vi "DET_get_Data_corrected.vi"(8 "error in (no error)":errorcluster, 10 "Control IN":T1={"# scans"=0, "All"=FALSE, "Parameters of measurement"={"ODmin"=0.0, "ODmax"=0.0, "Aq contol"=enum."fixed", "Wavelength_fix_index"=640, "WCM_limits"={"WCM_min"=0.0, "WCM_max"=0.0, "WCM_value"=0.0}, "WCM_corrections"=FALSE, "#cycles max"=5}}, 11 "Detector in":refnum<class "Detector.lvclass">) -> (0 "error out":errorcluster, 1 "II channel seq":cluster{"BG":i32[], "Ie":i32[], "I0":i32[]}[](array[cluster]), 2 "I channel seq":cluster{"BG":i32[], "Ie":i32[], "I0":i32[]}[](array[cluster]), 3 "Detector out":refnum<class "Detector.lvclass">, 5 "WCM_correction_coff":sgl[](array[numeric]))   [LabVIEW 2015, in "Detector.lvclass"]
uses:
  Detector.lvclass
  dependecies/ControlsVIs/Clusters-def/Det-Read.ctl
  dependecies/ControlsVIs/Clusters-def/Parameters_measurement_def.ctl
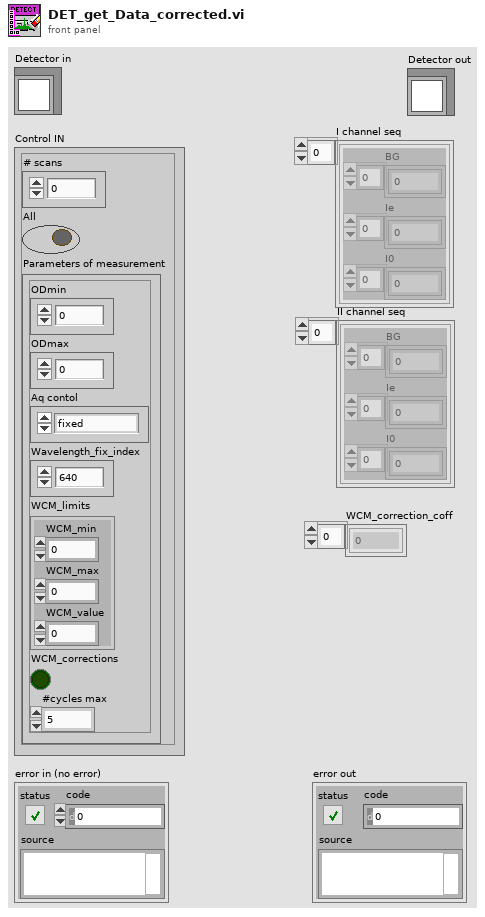
[diagram p1: front panel]
types:
  T1 = typedef "Detector.lvclass/Det-Read.ctl" = cluster{"# scans":i32, "All":bool, "Parameters of measurement":T2}
  T2 = typedef "Parameters_measurement_def.ctl" = cluster{"ODmin":dbl, "ODmax":dbl, "Aq contol":enum32{"fixed", "automatic", "fixed-auto"}, "Wavelength_fix_index":i32, "WCM_limits":cluster{"WCM_min":dbl, "WCM_max":dbl, "WCM_value":dbl}, "WCM_corrections":bool, "#cycles max":i32}
  T3 = cluster{"WCM_min":dbl, "WCM_max":dbl, "WCM_value":dbl}
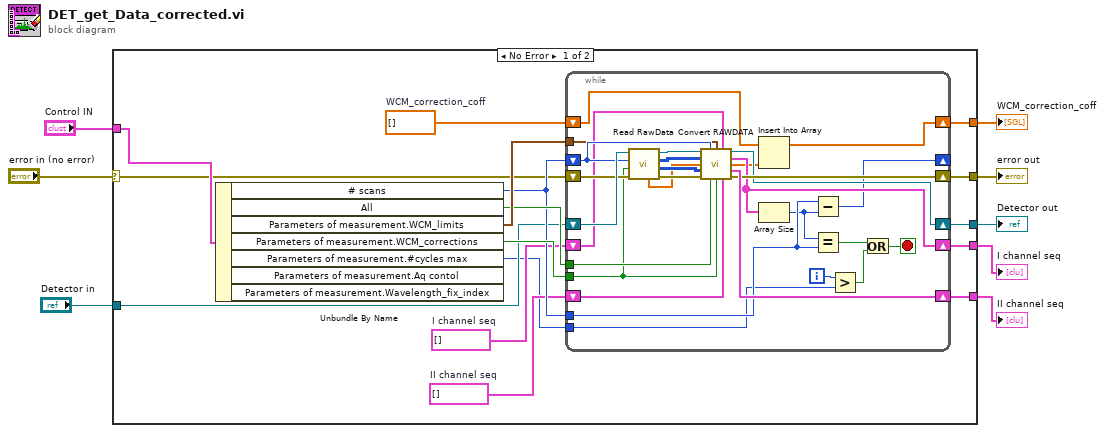
[diagram p0: block diagram]
diagram:
  n1 = case shown="No Error" "error in (no error)" {
    selector: "error in (no error)" -> [w10 w54]
    tunnel: [w18 _] -> w8
    tunnel: [w16 w53] -> w7
    tunnel: [w15 w54] -> w6
    tunnel: [w14 _] -> w5
    tunnel: [w13 _] -> w4
    tunnel: "Detector in" -> [w12 w53]
    tunnel: "Control IN" -> [w11 _]
    frame No Error {
      w20 = cluster{"BG":i32[], "Ie":i32[], "I0":i32[]}[] []  # II channel seq
      w19 = cluster{"BG":i32[], "Ie":i32[], "I0":i32[]}[] []  # I channel seq
      w17 = sgl[] []  # WCM_correction_coff
      n2 = Unbundle By Name(w11) -> ("# scans"=w21:i32, "All"=w22:bool, "Parameters of measurement.WCM_limits"=w23:T3, "Parameters of measurement.WCM_corrections"=w24:bool, "Parameters of measurement.#cycles max"=w9:i32)  [unwired: 2 out]
      n3 = while {
        shift-right: [w45] -> w16
        shift-left: w12 -> [w52]
        shift-right: [w46] -> w15
        shift-left: w10 -> [w44]
        shift-right: [w29] -> w18
        shift-left: w17 -> [w27]
        shift-right: [w40] -> w13
        shift-left: w19 -> [w42]
        shift-right: [w47] -> w14
        shift-left: w20 -> [w41]
        shift-right: [w33] -> _
        shift-left: w21 -> [w43]
        tunnel: w21 -> [w35]
        tunnel: w22 -> [w32]
        tunnel: w23 -> [w31]
        tunnel: w24 -> [w26]
        tunnel: w9 -> [w25]
        i -> [w39]
        stop <- w36 stop-if-true
        n4 = call-dynamic "Read RawData.vi"("error in (no error)"=w44, "WCM_max_value"=w26, "# of scans"=w43, "Detector in"=w52) -> ("error out"=w50:errorcluster, "Channel II"=w48:i32[][], "Channel I"=w49:i32[][], "Detector out"=w51:refnum<class "Detector.lvclass">, "WCM_values"=w30:sgl[])  [unwired: 3 in]
        n5 = call-dynamic "Convert RAWDATA.vi"("Detector in"=w51, "# of scan"=w43, "WCM_limits"=w31, "I channel seq IN"=w42, "I channel"=w49, "WCM_values IN"=w30, "II channel"=w48, "error in (no error)"=w50, "All?"=w32, "WCM_corrections"=w26, "II channel seq IN"=w41) -> ("Detector out"=w45:refnum<class "Detector.lvclass">, "I channel seq"=w40:cluster{"BG":i32[], "Ie":i32[], "I0":i32[]}[], "WCM_correction_coff"=w28:sgl[], "II channel seq"=w47:cluster{"BG":i32[], "Ie":i32[], "I0":i32[]}[], "error out"=w46:errorcluster)
        n6 = Insert Into Array(array=w27, new element=w28) -> (w29:sgl[])  [unwired: 1 in]
        n7 = Array Size(array=w40) -> (size(s)=w34:i32)
        n8 = Subtract(x=w35, y=w34) -> (x-y=w33:i32)
        n9 = Equal?(x=w34, y=w35) -> (x = y?=w38:bool)
        n10 = Greater?(x=w39, y=w25) -> (0:w37:bool)
        n11 = Or(x=w38, y=w37) -> (x .or. y?=w36:bool)
      }
    }
    frame Error {
    }
  }
  "WCM_correction_coff" <- w8
  "Detector out" <- w7
  "error out" <- w6
  "II channel seq" <- w5
  "I channel seq" <- w4
